vi "Drive.vi"(8 "Time":T1, 9 "Right Speed":T10, 10 "Left Speed":T10, 11 "RobotDriveDevRef":T2) -> (3 "RobotDriveDevRef 2":T2)   [LabVIEW 2015]
uses:
  <vilib>/Rock Robotics/WPI/RobotDrive/WPI_RobotDriveDevRef.ctl
  <vilib>/Rock Robotics/WPI/MotorControl/WPI_MotorControlDeviceRef.ctl
  <vilib>/Rock Robotics/WPI/MotorControl/WPI_MotorControlType.ctl
  <vilib>/Rock Robotics/SystemInterfaces/DIO/FPGA_DIOPWMChannel.ctl
  <vilib>/Rock Robotics/WPI/PWM/WPI_PWMDeadband.ctl
  <vilib>/Rock Robotics/WPI/CAN/Jaguar/SubVIs/WPI_CANJaguar_ControlMode.ctl
  <vilib>/Rock Robotics/WPI/CAN/TalonSRX/WPI_CANTalonSRX_APIControlMode.ctl
  Controls/Speed.ctl
  Controls/Time.ctl
panel:
  out "Numeric 2":dbl
  out "Numeric":dbl
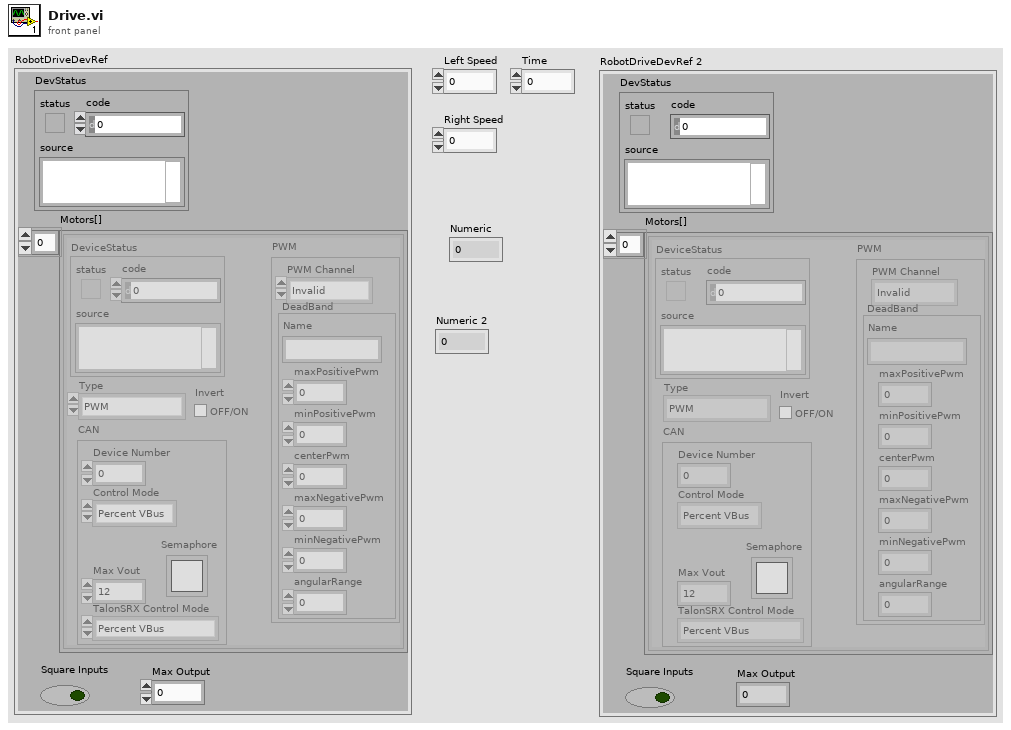
[diagram p1: front panel]
types:
  T1 = typedef "Time.ctl" = dbl
  T2 = typedef "WPI_RobotDriveDevRef.ctl" = cluster{"DevStatus":errorcluster, "Motors[]":T3[], "Square Inputs":bool, "Max Output":dbl}
  T3 = typedef "WPI_MotorControlDeviceRef.ctl" = cluster{"DeviceStatus":errorcluster, "Type":T4, "PWM":cluster{"PWM Channel":T5, "DeadBand":T6}, "CAN":cluster{"Device Number":u8, "Control Mode":T7, "Semaphore":T8, "Max Vout":dbl, "TalonSRX Control Mode":T9}, "Invert":bool}
  T4 = typedef "WPI_MotorControlType.ctl" = enum16{"PWM", "CAN", "CANTalonSRX"}
  T5 = typedef "FPGA_DIOPWMChannel.ctl" = enum8{"PWM 0", "PWM 1", "PWM 2", "PWM 3", "PWM 4", "PWM 5", "PWM 6", "PWM 7", "PWM 8", "PWM 9", "PWM MXP 0", "PWM MXP 1", "PWM MXP 2", "PWM MXP 3", "PWM MXP 4", "PWM MXP 5", "PWM MXP 6", "PWM MXP 7", "PWM MXP 8", "PWM MXP 9", "Invalid"}
  T6 = typedef "WPI_PWMDeadband.ctl" = cluster{"Name":string, "maxPositivePwm":i32, "minPositivePwm":i32, "centerPwm":i32, "maxNegativePwm":i32, "minNegativePwm":i32, "angularRange":u16}
  T7 = typedef "WPI_CANJaguar_ControlMode.ctl" = enum8{"Percent VBus", "Current", "Speed", "Position", "Voltage"}
  T8 = typedef "Semaphore RefNum" = refnum<k1>
  T9 = typedef "WPI_CANTalonSRX_APIControlMode.ctl" = enum8{"Percent VBus", "Speed", "Position", "Slave", "Unchanged / Invalid", "Voltage Compensation", "Current", "Motion Profile"}
  T10 = typedef "Speed.ctl" = dbl
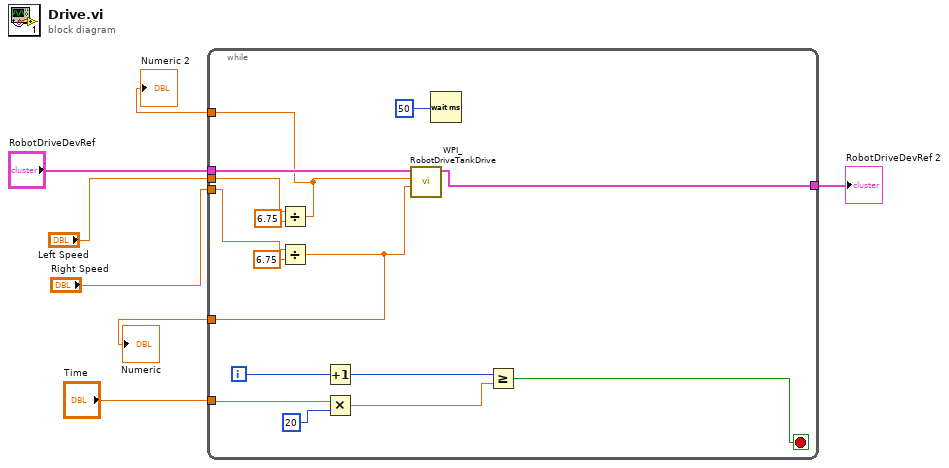
[diagram p0: block diagram]
diagram:
  n1 = while {
    tunnel: "RobotDriveDevRef" -> [w22]
    tunnel: "Left Speed" -> [w13]
    tunnel: "Time" -> [w17]
    tunnel: "Right Speed" -> [w11]
    tunnel: [w14] -> w4
    tunnel: [w9] -> w2
    tunnel: [w8] -> w1
    i -> [w20]
    stop <- w18 stop-if-true
    n2 = Divide(x=w13, y=6.75) -> (x/y=w9:T10)
    n3 = Divide(x=w11, y=6.75) -> (x/y=w8:T10)
    n4 = Increment(x=w20) -> (x+1=w19:i32)
    n5 = Multiply(x=w17, y=20) -> (x*y=w16:T1)
    n6 = call <vilib>:"WPI_RobotDriveTankDrive.vi"("Right axis value"=w8, "Left axis value"=w9, "RobotDriveDevRef"=w22) -> ("RobotDriveDevRef"=w14:T2)  [unwired: 6 in, 2 out]
    n7 = Wait (ms)(milliseconds to wait=50) -> ()  [unwired: 1 out]
    n8 = Greater Or Equal?(x=w19, y=w16) -> (x >= y?=w18:bool)
  }
  "RobotDriveDevRef 2" <- w4
  "Numeric 2" <- w2
  "Numeric" <- w1
